vi "stop.vi"() -> (2 "Boolean":bool)   [LabVIEW 2017]
uses:
  <vilib>/Rock Robotics/WPI/DriverStation/WPI_DriverStationRobotMode2.ctl
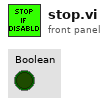
[diagram p1: front panel]
types:
  T1 = typedef "WPI_DriverStationRobotMode2.ctl" = enum16{"Autonomous Disabled", "Autonomous Enabled", "Teleop Disabled", "Teleop Enabled", "Disconnected", "Finish", "Test Disabled", "Test Enabled", "Emergency Stopped"}
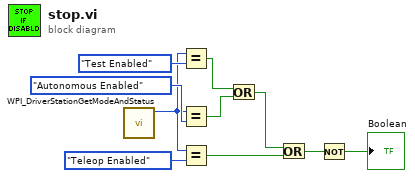
[diagram p0: block diagram]
diagram:
  n1 = call <vilib>:"WPI_DriverStationGetModeAndStatus.vi"() -> ("Robot Mode"=w7:T1)  [unwired: 10 in, 1 out]
  n2 = Equal?(x=w7, y=WPI_DriverStationRobotMode2."Test Enabled") -> (x = y?=w6:bool)
  n3 = Equal?(x=w7, y=WPI_DriverStationRobotMode2."Autonomous Enabled") -> (x = y?=w5:bool)
  n4 = Equal?(x=w7, y=WPI_DriverStationRobotMode2."Teleop Enabled") -> (x = y?=w3:bool)
  n5 = Or(x=w6, y=w5) -> (x .or. y?=w4:bool)
  n6 = Or(x=w4, y=w3) -> (x .or. y?=w2:bool)
  n7 = Not(x=w2) -> (.not. x?=→"Boolean":bool)
